vi "FPGA_Qudi_Scan_trigger_camera_synchro_laser_lines.vi"(3 "N Z positions":i32) -> ()   [LabVIEW 2015]
uses:
  <vilib>/rvi/Analysis/control/PID/Typedef/niFpgaPID_PIGains.ctl
  <vilib>/Platform/TimedLoop/XDataNode/timing_clust.ctl
  <vilib>/Platform/TimedLoop/XDataNode/nitl_modes.ctl
  <vilib>/Platform/TimedLoop/XDataNode/wakeup.ctl
  <vilib>/rvi/FXPMathLib/basic elements/FxpIntAccumulator/subVIs/nifxpmath_IntAccumulator_SimConfig.ctl
  <vilib>/rvi/Emulation/niFpgaGetClockAttributes.vi
  <vilib>/rvi/Emulation/niFpgaSctlEmulationGetInTimedLoop.vi
  <vilib>/rvi/Emulation/niFpgaEmulationReportErrorSimple.vi
  <vilib>/rvi/eio/common/nirviEmuTemplateMethod_errors.vi
  <vilib>/rvi/Emulation/niFpgaCriticalErrorInLSC.vi
  <vilib>/rvi/Emulation/niFpgaProcessEmulError.vi
  <vilib>/rvi/Analysis/common/codeGenErrors/XNode/niFpgaXNodeCodeGenErrorHandle.vi
  <vilib>/rvi/FXPMathLib/basic elements/FxpIntAccumulator/simVIs/DllFxpIntAccumulator_sub.vi
  <vilib>/rvi/Analysis/control/PID/SubVIs/niFpgaPID_PIWrapper.vi
  <vilib>/eio/EIONode/EIONode.xnode
  <vilib>/rvi/Analysis/measure/dc-rms/XNode/niFpgaDC-RMS.xnode
  <vilib>/Platform/TimedLoop/XDataNode/XDataNode.xnode
  <vilib>/rvi/FXPMathLib/basic elements/FxpIntAccumulator/XNode/nifxpmath_IntAccumulator.xnode
  <vilib>/Platform/TimedLoop/XDataNode/XDNodeRunTimeDep.lvlib
panel:
  in  "integration_time_us":u32=100 caption="Count(uSec)"
  in  "stop":bool
  out "duration_ms":u32
  out "X":i16
  out "Y":i16
  out "Sum":i16
  out "counter":u32
  out "output":i16
  in  "reset":bool
  in  "reset_counter":bool
  in  "autofocus":bool
  in  "setpoint":i16
  in  "P":i16
  in  "I":i16
  in  "ref_axis":bool
  out "Images acquired":i32
  in  "Laser lines":i32[](array[numeric])=[0, 0, 0, 0, 0]
  in  "Laser power":i16[](array[numeric])=[0, 0, 0, 0, 0]
  in  "N laser lines":i32
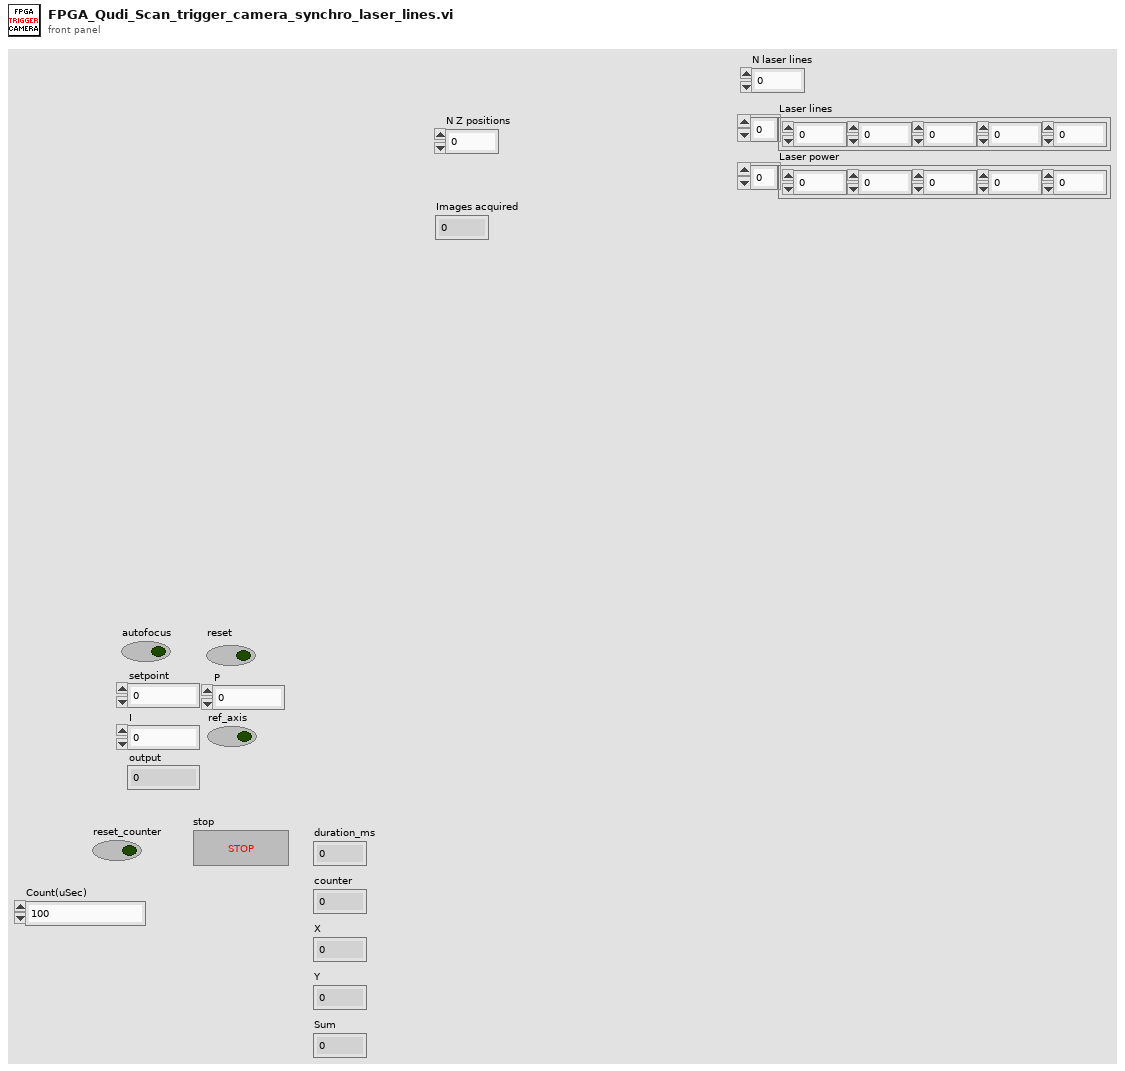
[diagram p1: front panel]
types:
  T1 = typedef "niFpgaPID_PIGains.ctl" = cluster{"proportional gain":sgl, "integral gain":sgl}
  T2 = typedef "XDNodeRunTimeDep.lvlib/timing_clust.ctl" = cluster{"Expected End [f-1]":u64, "Actual End [f-1]":u64, "Finished Late? [f-1]":bool, "Expected End [i-1]":u64, "Actual End [i-1]":u64, "Finished Late? [i-1]":bool, "Expected Start [i]":u64, "Actual Start [i]":u64, "Expected Start [f]":u64, "Actual Start [f]":u64, "Source Name":string, "Structure Name":string, "Period":i64, "Deadline":i64, "Offset":i64, "Start":i64, "Priority":i32, "Timeout":i32, "Mode":T3, "Wakeup Reason":T4, "Error":errorcluster, "Source Type":string, "Secondary Source Type":string, "Global End Time":u64, "Global Start Time":u64, "Frame Duration":u64, "Iteration Duration":u64, "Assigned CPU":i32, "I/O Scan Engine Mode":u32}
  T3 = typedef "XDNodeRunTimeDep.lvlib/nitl_modes.ctl" = enum32{"No Change", "Process missed periods, maintain original phase", "Discard missed periods, maintain original phase", "Process missed periods, ignore original phase", "Discard missed periods, ignore original phase"}
  T4 = typedef "XDNodeRunTimeDep.lvlib/wakeup.ctl" = enum32{"Normal", "Aborted", "Asynchronous wakeup", "Timing source error", "Timed loop error", "Timeout"}
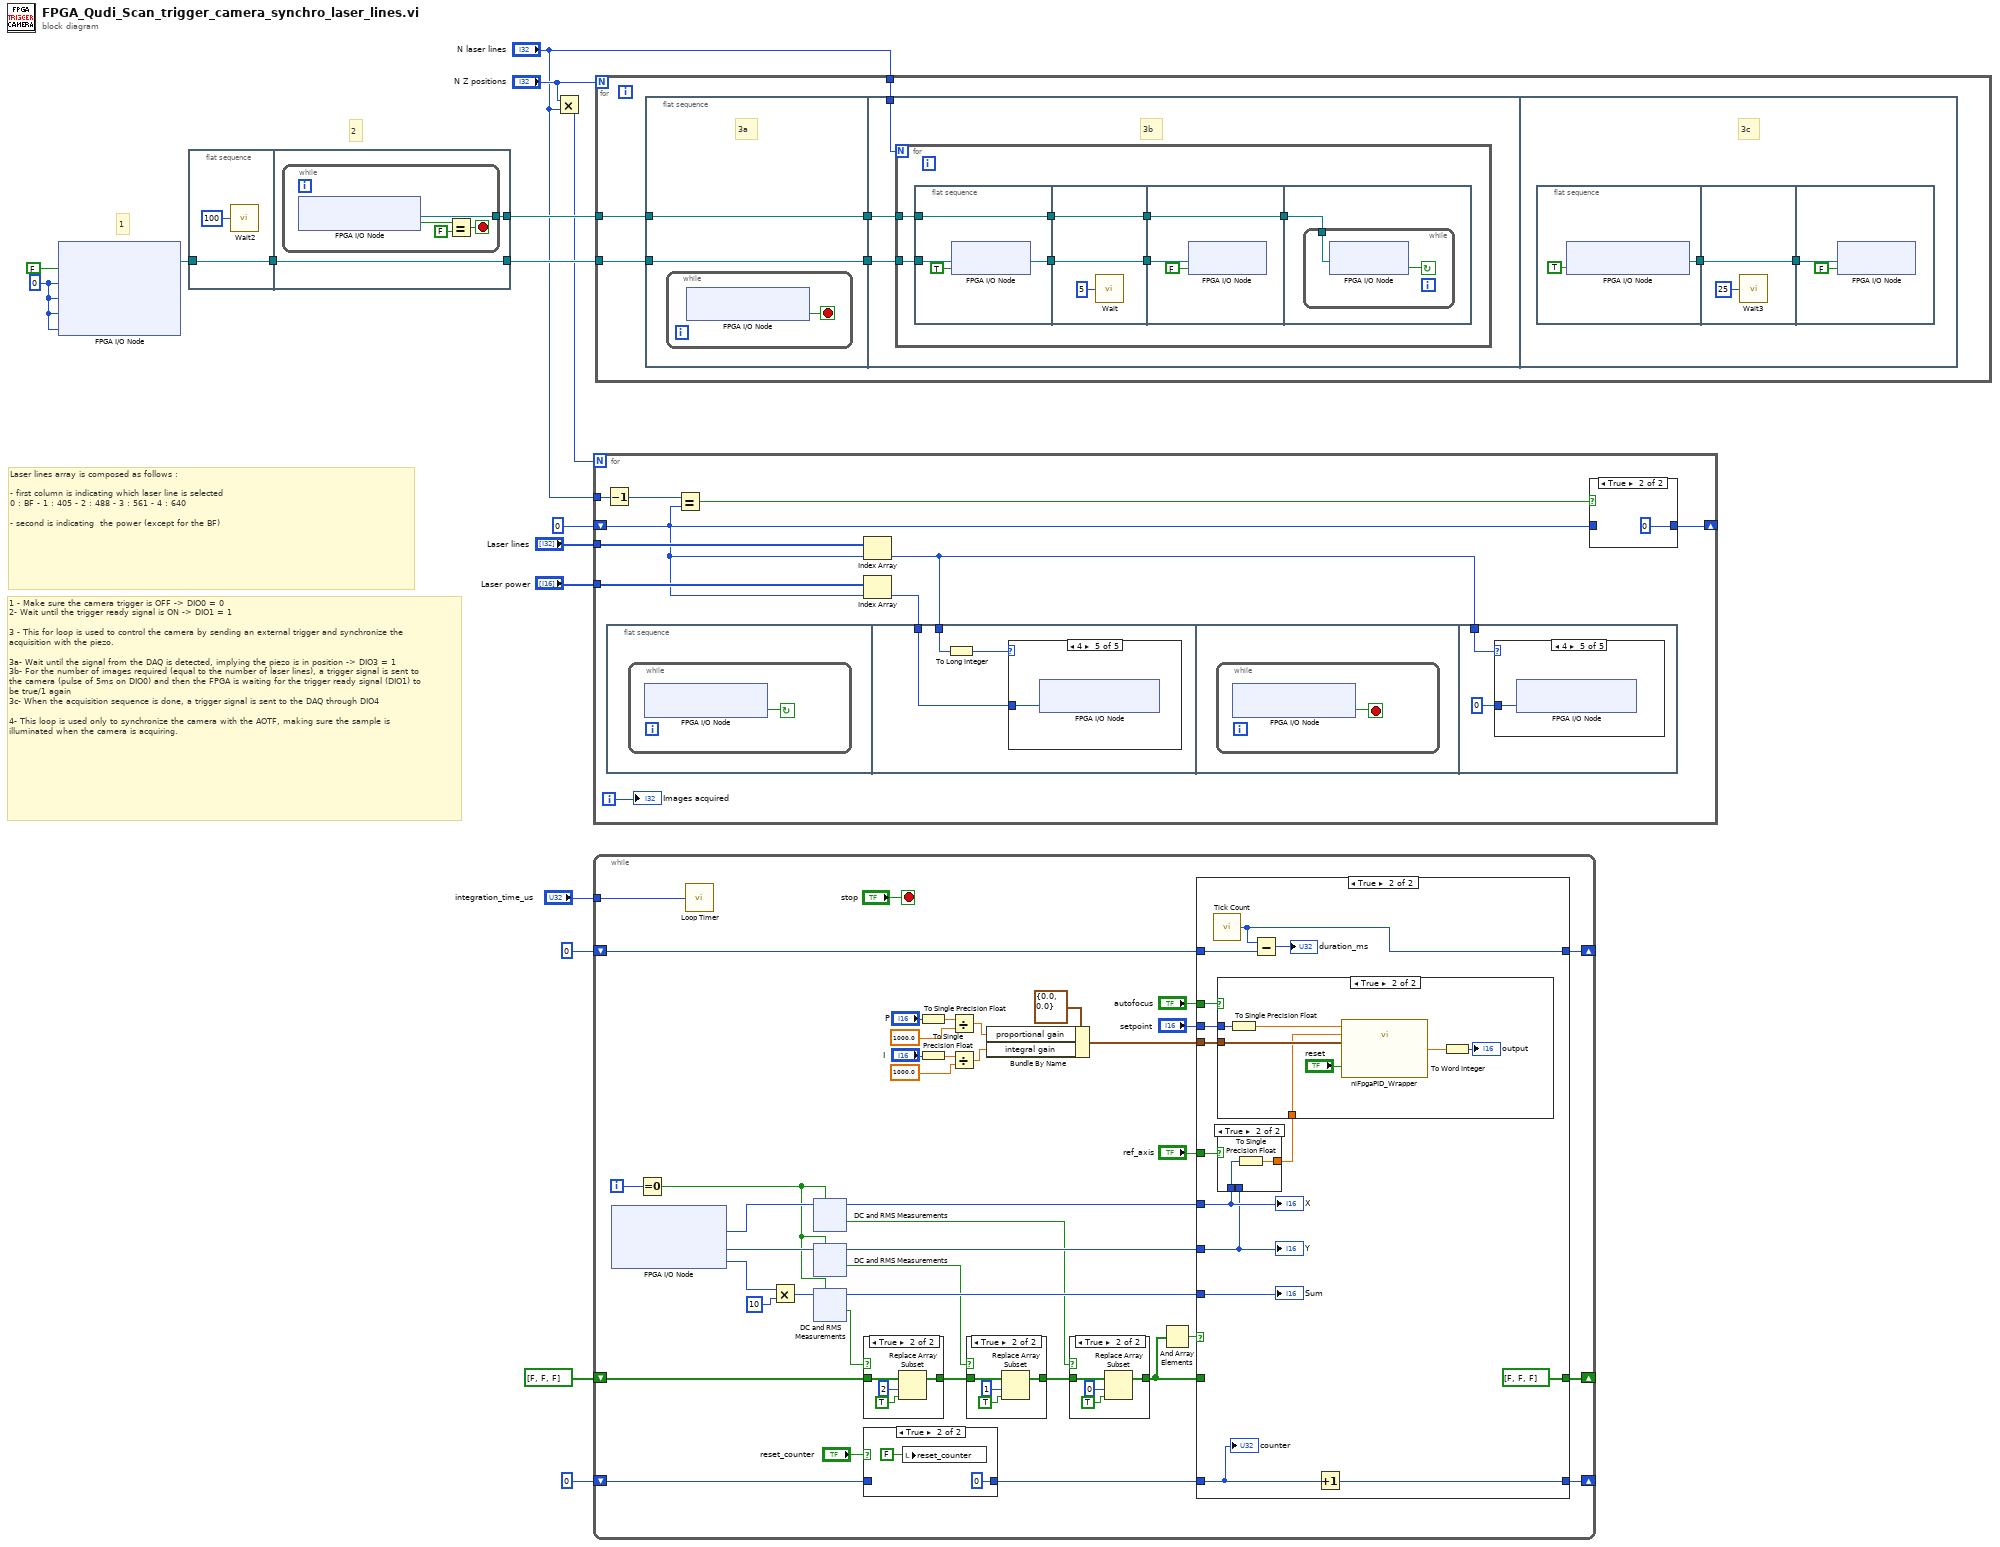
[diagram p0: block diagram]
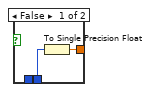
[diagram p7: hidden frame]
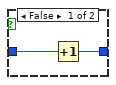
[diagram p9: hidden frame]
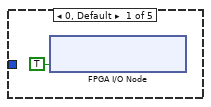
[diagram p10: hidden frame]
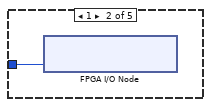
[diagram p11: hidden frame]
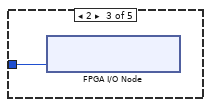
[diagram p12: hidden frame]
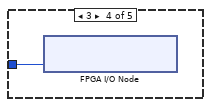
[diagram p13: hidden frame]
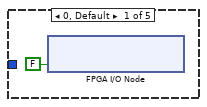
[diagram p14: hidden frame]
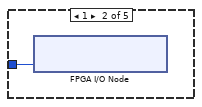
[diagram p15: hidden frame]
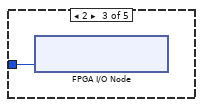
[diagram p16: hidden frame]
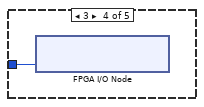
[diagram p17: hidden frame]
diagram:
  w5 = i16 0 ("Connector0/AO0")
  # "2"
  # "1"
  # "1 - Make sure the camera trigger is OFF -> DIO0 = 0\n2- Wait until the trigger ready signal is ON -> DIO1 = 1\n\n3 - This for loop is used to control the camera by sending an external trigger and synchronize the acquisition with the piezo.\n\n3a- Wait until the signal from the DAQ is detected, implying the piezo is in position -> DIO3 = 1 \n3b- For the number of images required (equal to the number of laser lines), a trigger signal is sent to the camera (pulse of 5ms on DIO0) and then the FPGA is waiting for the trigger ready signal (DIO1) to be true/1 again\n3c- When the acquisition sequence is done, a trigger signal is sent to the DAQ through DIO4\n\n4- This loop is used only to synchronize the camera with the AOTF, making sure the sample is illuminated when the camera is acquiring."
  # "Laser lines array is composed as follows :\n\n- first column is indicating which laser line is selected \n0 : BF - 1 : 405 - 2 : 488 - 3 : 561 - 4 : 640\n\n- second is indicating  the power (except for the BF)"
  n1 = xnode "FPGA I/O Node"("Connector0/DIO0"=FALSE, "Connector0/AO0"=w5, "Connector0/AO1"=w5, "Connector0/AO2"=w5, "Connector0/AO3"=w5) -> ("FPGA I/O Out"=w15:refnum<k21>)  [unwired: 5 in, 4 out]
  n2 = flat-sequence {
    tunnel: w15 -> [w18]
    tunnel: [w18] -> w14
    tunnel: w14 -> [w20]
    tunnel: [w20] -> w13
    tunnel: [w19] -> w12
    frame #0 {
      n3 = call "Wait2"("Count(uSec)"=u32 100 ("Count(mSec)")) -> ()  [unwired: 1 out]
    }
    frame #1 {
      n4 = while {
        tunnel: [w24] -> w19
        stop <- w21 stop-if-true
        n5 = xnode "FPGA I/O Node"() -> ("Connector0/DIO1"=w23:bool, "FPGA I/O Out"=w24:refnum<k21>)  [unwired: 1 in]
        n6 = Equal?(x=w23, y=FALSE) -> (x = y?=w21:bool)
      }
    }
  }
  n7 = Multiply(x="N Z positions", y="N laser lines") -> (x*y=w7:i32)
  n8 = for {
    N: w7 -> [_]
    shift-right: [w32] -> _
    shift-left: 0 -> [w29]
    tunnel: "Laser lines" -> [w31]
    tunnel: "Laser power" -> [w30]
    tunnel: "N laser lines" -> [w27]
    i -> [w25]
    n9 = Decrement(x=w27) -> (x-1=w26:i32)
    n10 = flat-sequence {
      tunnel: w34 -> [w40]
      tunnel: w28 -> [w39]
      tunnel: w34 -> [w48]
      frame #0 {
        n11 = while {
          stop <- w38 continue-if-true
          n12 = xnode "FPGA I/O Node"() -> ("Connector0/DIO2"=w38:bool)  [unwired: 1 in, 1 out]
        }
      }
      frame #1 {
        n13 = To Long Integer(number=w40) -> (32bit integer=w41:i32)
        n14 = case shown="4" w41 {
          tunnel: w39 -> [_ w43 w44 w45 w46]
          frame 0, Default {
            n15 = xnode "FPGA I/O Node"("Connector0/DIO5"=TRUE) -> ()  [unwired: 1 in, 1 out]
          }
          frame 1 {
            n16 = xnode "FPGA I/O Node"("Connector0/AO2"=w43) -> ()  [unwired: 1 in, 1 out]
          }
          frame 2 {
            n17 = xnode "FPGA I/O Node"("Connector0/AO3"=w44) -> ()  [unwired: 1 in, 1 out]
          }
          frame 3 {
            n18 = xnode "FPGA I/O Node"("Connector0/AO0"=w45) -> ()  [unwired: 1 in, 1 out]
          }
          frame 4 {
            n19 = xnode "FPGA I/O Node"("Connector0/AO1"=w46) -> ()  [unwired: 1 in, 1 out]
          }
        }
      }
      frame #2 {
        n20 = while {
          stop <- w47 stop-if-true
          n21 = xnode "FPGA I/O Node"() -> ("Connector0/DIO2"=w47:bool)  [unwired: 1 in, 1 out]
        }
      }
      frame #3 {
        n22 = case shown="4" w48 {
          tunnel: i16 0 -> [_ w51 w52 w53 w54]
          frame 0, Default {
            n23 = xnode "FPGA I/O Node"("Connector0/DIO5"=FALSE) -> ()  [unwired: 1 in, 1 out]
          }
          frame 1 {
            n24 = xnode "FPGA I/O Node"("Connector0/AO2"=w51) -> ()  [unwired: 1 in, 1 out]
          }
          frame 2 {
            n25 = xnode "FPGA I/O Node"("Connector0/AO3"=w52) -> ()  [unwired: 1 in, 1 out]
          }
          frame 3 {
            n26 = xnode "FPGA I/O Node"("Connector0/AO0"=w53) -> ()  [unwired: 1 in, 1 out]
          }
          frame 4 {
            n27 = xnode "FPGA I/O Node"("Connector0/AO1"=w54) -> ()  [unwired: 1 in, 1 out]
          }
        }
      }
    }
    n28 = Equal?(x=w26, y=w29) -> (x = y?=w33:bool)
    n29 = Index Array(array=w31, index=w29) -> (element=w34:i32)
    n30 = Index Array(array=w30, index=w29) -> (element=w28:i16)
    n31 = case shown="True" w33 {
      tunnel: w29 -> [w36 _]
      tunnel: [w35 0] -> w32
      frame False {
        n32 = Increment(x=w36) -> (x+1=w35:i32)
      }
      frame True {
      }
    }
    "Images acquired" <- w25
  }
  n33 = while {
    shift-right: [w78] -> _
    shift-left: bool[] [FALSE, FALSE, FALSE] ("initialized array") -> [w86]
    shift-right: [w76] -> _
    shift-left: u32 0 -> [w77]
    tunnel: "integration_time_us" -> [w75]
    shift-right: [w74] -> _
    shift-left: u32 0 -> [w72]
    i -> [w92]
    stop <- "stop" stop-if-true
    n34 = xnode "FPGA I/O Node"() -> ("Connector0/AI0"=w94:i16, "Connector0/AI1"=w90:i16, "Connector0/AI2"=w57:i16)  [unwired: 3 in, 3 out]
    n35 = Equal To 0?(x=w92) -> (x = 0?=w87:bool)
    n36 = call "Loop Timer"("Count(uSec)"=w75) -> ()  [unwired: 1 out]
    n37 = Multiply(x=w57, y=i16 10) -> (x*y=w56:i16)
    n38 = xnode "DC and RMS Measurements"("input data"=w94, "reset"=w87) -> ("DC"=w91:i16, "output valid"=w81:bool)
    n39 = xnode "DC and RMS Measurements"("input data"=w90, "reset"=w87) -> ("DC"=w89:i16, "output valid"=w82:bool)
    n40 = xnode "DC and RMS Measurements"("input data"=w56, "reset"=w87) -> ("DC"=w88:i16, "output valid"=w83:bool)
    n41 = case shown="True" w83 {
      tunnel: w86 -> [w103 w106]
      tunnel: [w103 w104] -> w85
      frame False {
      }
      frame True {
        n42 = Replace Array Subset(array=w106, new element=TRUE, index=2) -> (w104:bool[])
      }
    }
    n43 = case shown="True" "reset_counter" {
      tunnel: w72 -> [w95 _]
      tunnel: [w95 u32 0] -> w71
      frame False {
      }
      frame True {
        n44 = local write "reset_counter"(FALSE ("Reset counter")) -> ()
      }
    }
    n45 = To Single Precision Float(number="P") -> (single precision float=w64:sgl)
    n46 = To Single Precision Float(number="I") -> (single precision float=w61:sgl)
    n47 = Divide(x=w64, y=sgl 1000.0) -> (x/y=w62:sgl)
    n48 = Divide(x=w61, y=sgl 1000.0) -> (x/y=w59:sgl)
    n49 = case shown="True" w82 {
      tunnel: w85 -> [w108 w111]
      tunnel: [w108 w109] -> w84
      frame False {
      }
      frame True {
        n50 = Replace Array Subset(array=w111, new element=TRUE, index=1) -> (w109:bool[])
      }
    }
    n51 = Bundle By Name(cluster=T1 {"proportional gain"=0.0, "integral gain"=0.0} ("gains"), "proportional gain"=w62, "integral gain"=w59) -> (w65:T1)
    n52 = case shown="True" w81 {
      tunnel: [w98 w100] -> w79
      tunnel: w84 -> [w98 w99]
      frame False {
      }
      frame True {
        n53 = Replace Array Subset(array=w99, new element=TRUE, index=0) -> (w100:bool[])
      }
    }
    n54 = And Array Elements(Boolean array=w79) -> (logical AND=w80:bool)
    n55 = case shown="True" w80 {
      tunnel: w91 -> [_ w118]
      tunnel: w89 -> [_ w116]
      tunnel: w88 -> [_ w124]
      tunnel: w79 -> [w115 _]
      tunnel: [w115 bool[] [FALSE, FALSE, FALSE] ("initialized array")] -> w78
      tunnel: w77 -> [w114 w128]
      tunnel: [w114 w126] -> w76
      tunnel: w71 -> [w113 w123]
      tunnel: [w113 w125] -> w74
      tunnel: "autofocus" -> [_ w122]
      tunnel: "setpoint" -> [_ w121]
      tunnel: w65 -> [_ w120]
      tunnel: "ref_axis" -> [_ w119]
      frame False {
      }
      frame True {
        n56 = call "Tick Count"() -> ("Tick Count(mSec)"=w126:u32)
        n57 = case shown="True" w119 {
          tunnel: w118 -> [_ w133]
          tunnel: [w130 w132] -> w117
          tunnel: w116 -> [w131 _]
          frame False {
            n58 = To Single Precision Float(number=w131) -> (single precision float=w130:sgl)
          }
          frame True {
            n59 = To Single Precision Float(number=w133) -> (single precision float=w132:sgl)
          }
        }
        n60 = case shown="True" w122 {
          tunnel: w121 -> [_ w140]
          tunnel: w120 -> [_ w138]
          tunnel: w117 -> [_ w134]
          frame False {
          }
          frame True {
            n61 = To Single Precision Float(number=w140) -> (single precision float=w139:sgl)
            n62 = call-poly <vilib>:"niFpgaPID_Wrapper.vi"("setpoint"=w139, "reset? (F)"="reset", "process variable"=w134, "gains"=w138) -> ("output"=w136:sgl)  [unwired: 9 in, 2 out]
            n63 = To Word Integer(number=w136) -> (16bit integer=→"output":i16)
          }
        }
        n64 = Subtract(x=w126, y=w128) -> (x-y=→"duration_ms":u32)
        n65 = Increment(x=w123) -> (x+1=w125:u32)
        "X" <- w118
        "Y" <- w116
        "Sum" <- w124
        "counter" <- w123
      }
    }
  }
  n66 = for {
    N: "N Z positions" -> [_]
    tunnel: w13 -> [w399]
    tunnel: w12 -> [w400]
    tunnel: "N laser lines" -> [w396]
    n67 = flat-sequence {
      tunnel: w399 -> [w401]
      tunnel: w400 -> [w402]
      tunnel: [w402] -> w398
      tunnel: [w401] -> w397
      tunnel: w398 -> [w406]
      tunnel: w397 -> [w405]
      tunnel: w396 -> [w404]
      frame #0 {
        # "3a"
        n68 = while {
          stop <- w403 stop-if-true
          n69 = xnode "FPGA I/O Node"() -> ("Connector0/DIO3"=w403:bool)  [unwired: 1 in, 1 out]
        }
      }
      frame #1 {
        # "3b"
        n70 = for {
          N: w404 -> [_]
          tunnel: w406 -> [w408]
          tunnel: w405 -> [w407]
          n71 = flat-sequence {
            tunnel: [w416] -> w413
            tunnel: [w414] -> w412
            tunnel: w407 -> [w415]
            tunnel: w408 -> [w414]
            tunnel: w413 -> [w419]
            tunnel: [w419] -> w411
            tunnel: [w418] -> w410
            tunnel: w412 -> [w418]
            tunnel: w411 -> [w422]
            tunnel: [w421] -> w409
            tunnel: w410 -> [w421]
            tunnel: w409 -> [w424]
            frame #0 {
              n72 = xnode "FPGA I/O Node"("I/O Item"=TRUE ("Connector0/DIO0"), "FPGA I/O In"=w415) -> ("FPGA I/O Out"=w416:refnum<k21>)
            }
            frame #1 {
              n73 = call "Wait"("Count(mSec)"=u32 5) -> ()  [unwired: 1 out]
            }
            frame #2 {
              n74 = xnode "FPGA I/O Node"("I/O Item"=FALSE ("Connector0/DIO0"), "FPGA I/O In"=w422) -> ()  [unwired: 1 out]
            }
            frame #3 {
              n75 = while {
                tunnel: w424 -> [w426]
                stop <- w425 continue-if-true
                n76 = xnode "FPGA I/O Node"("FPGA I/O In"=w426) -> ("I/O Item"=w425:bool)  [unwired: 1 out]
              }
            }
          }
        }
      }
      frame #2 {
        # "3c"
        n77 = flat-sequence {
          tunnel: [w430] -> w428
          tunnel: w428 -> [w431]
          tunnel: [w431] -> w427
          tunnel: w427 -> [w433]
          frame #0 {
            n78 = xnode "FPGA I/O Node"("Connector0/DIO4"=TRUE) -> ("FPGA I/O Out"=w430:refnum<k21>)  [unwired: 1 in]
          }
          frame #1 {
            n79 = call "Wait3"("Count(mSec)"=u32 25) -> ()  [unwired: 1 out]
          }
          frame #2 {
            n80 = xnode "FPGA I/O Node"("I/O Item"=FALSE ("Connector0/DIO0"), "FPGA I/O In"=w433) -> ()  [unwired: 1 out]
          }
        }
      }
    }
  }
